vi "Motion-PollAxis-Main.vi"(8 "error in (no error)":errorcluster, 11 "Motion-ControlAll in":refnum<class "Motion-ControlAll.lvclass">) -> (0 "error out":errorcluster, 3 "Motion-ControlAll out":refnum<class "Motion-ControlAll.lvclass">)   [LabVIEW 2013, in "Motion-ControlAll.lvclass"]
uses:
  Motion-ControlAll.lvclass
  <vilib>/addons/_LabVIEW Style Book/Utilities/Style Book Utilities.lvlib
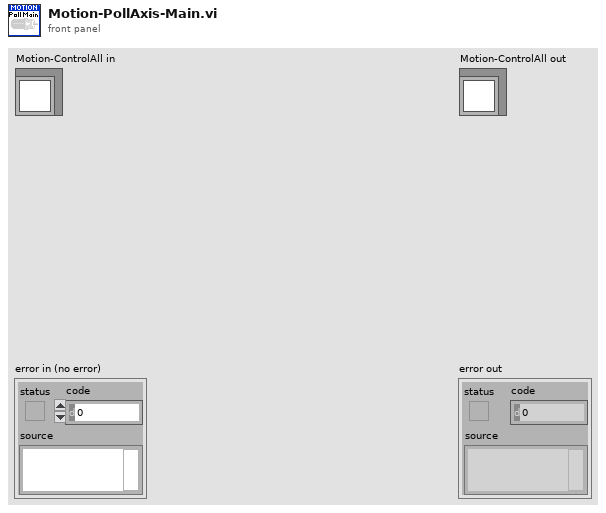
[diagram p1: front panel]
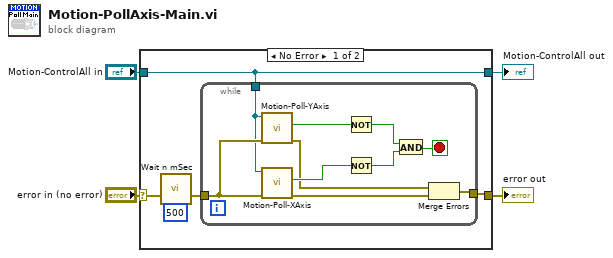
[diagram p0: block diagram]
diagram:
  n1 = case shown="No Error" "error in (no error)" {
    selector: "error in (no error)" -> [w7 w21]
    tunnel: [w8 w21] -> w3
    tunnel: [w9 w20] -> w1
    tunnel: "Motion-ControlAll in" -> [w9 w20]
    frame No Error {
      n2 = call <vilib>:"Wait n mSec.vi"("error in (no error)"=w7, "Milliseconds to Wait (500)"=u32 500) -> ("error out"=w6:errorcluster)  [unwired: 13 in]
      n3 = while {
        tunnel: w6 -> [w19]
        tunnel: w9 -> [w18]
        tunnel: [w10] -> w8
        stop <- w13 stop-if-true
        n4 = call "Motion-Poll-YAxis.vi"("error in (no error)"=w19, "Motion-ControlAll in"=w18) -> ("error out"=w11:errorcluster, "Y axis \nstopped"=w17:bool)  [unwired: 7 in, 1 out]
        n5 = call "Motion-Poll-XAxis.vi"("error in (no error)"=w19, "Motion-ControlAll in"=w18) -> ("error out"=w12:errorcluster, "X axis \nstopped"=w16:bool)  [unwired: 7 in, 1 out]
        n6 = Not(x=w17) -> (.not. x?=w14:bool)
        n7 = Not(x=w16) -> (.not. x?=w15:bool)
        n8 = And(x=w14, y=w15) -> (x .and. y?=w13:bool)
        n9 = Merge Errors(w11, w12) -> (w10:errorcluster)
      }
    }
    frame Error {
    }
  }
  "error out" <- w3
  "Motion-ControlAll out" <- w1
